vi "DAQmx Write (Digital 1D Bool NChan 1Samp 1Line).vi"(0 "task/channels in":refnum<k21>, 1 "auto start":bool=TRUE, 7 "data":bool[](array[boolean]), 9 "timeout":dbl=10.0 format="%0.2f", 11 "error in":errorcluster) -> (4 "task out":refnum<k21>, 10 "number of samples written per channel":u32, 15 "error out":errorcluster)   [LabVIEW 2013]
doc: "Writes a single sample of Boolean values to each channel in a task that contains multiple digital output channels. Each channel in the task can contain only one digital line."
uses:
  nilvaiu.dll
panel:
  # "channel"
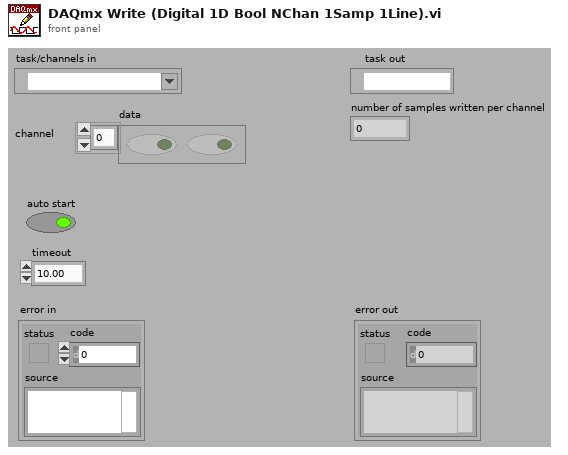
[diagram p1: front panel]
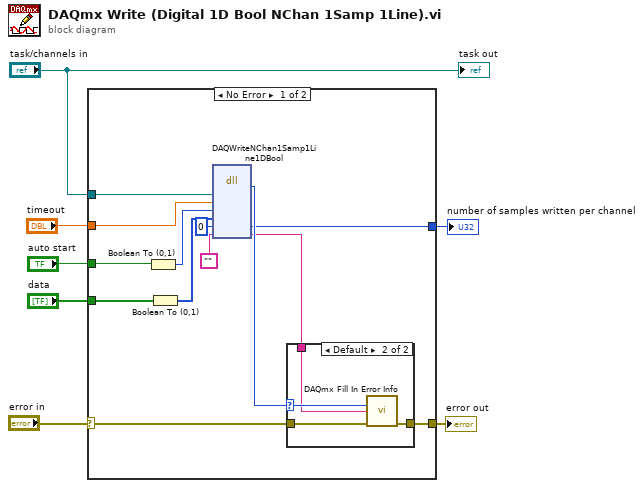
[diagram p0: block diagram]
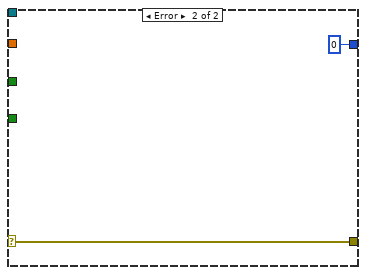
[diagram p3: hidden frame]
diagram:
  n1 = case shown="No Error" "error in" {
    selector: "error in" -> [w19 w27]
    tunnel: [w20 w27] -> w6
    tunnel: "task/channels in" -> [w18 _]
    tunnel: [w11 u32 0 ("numSamplesWriten")] -> w4
    tunnel: "timeout" -> [w10 _]
    tunnel: "auto start" -> [w9 _]
    tunnel: "data" -> [w8 _]
    frame No Error {
      n2 = Boolean To (0,1)(Boolean=w9) -> (0, 1=w15:i16)
      n3 = Boolean To (0,1)(Boolean=w8) -> (0, 1=w12:i16[])
      n4 = dll-call lib="nilvaiu.*" fn="DAQWriteNChan1Samp1Line1DBool"("taskID"=w18, "timeout"=w10, "autoStart"=w15, "data"=w12, "numSamplesWriten"=u32 0, "extendedErrorInfo"="") -> (w17:i32, "numSamplesWriten"=w11:u32, "extendedErrorInfo"=w14:string)  [unwired: 4 in, 5 out]
      n5 = case shown="Default" w17 {
        selector: w17 -> [_ w23]
        tunnel: w19 -> [w21 w25]
        tunnel: [w21 w24] -> w20
        tunnel: w14 -> [_ w22]
        frame 0 {
        }
        frame Default {
          n6 = call "DAQmx Fill In Error Info.vi"("status code"=w23, "extended error info"=w22, "error in"=w25) -> ("error out"=w24:errorcluster)  [unwired: 1 in, 11 out]
        }
      }
    }
    frame Error {
    }
  }
  "error out" <- w6
  "number of samples written per channel" <- w4
  "task out" <- "task/channels in"
